vi "CAN_Write_Read_NEW.vi"(5 "Read In":refnum<k21>, 7 "Numeric Request":u32, 8 "CAN frame":T1 {"payload" format="%x"; "timestamp" format="%<%.7X\n%x>T"; "type" items=["CAN Data"=0, "CAN Remote"=1, "CAN Bus Error"=2, "CAN 2.0 Data"=8, "CAN FD Data"=16, "CAN FD+BRS Data"=24, "J1939 Data"=192, "Delay"=224, "Log Trigger"=225, "Start Trigger"=226]; "identifier" format="%x"}, 9 "Write In":refnum<k21>) -> (0 "Error Out":errorcluster, 1 "cluster":T3 {"data[0]"."payload" format="%x"; "data[0]"."timestamp" format="%<%.7X\n%x>T"; "data[0]"."type" items=["CAN Data"=0, "CAN Remote"=1, "CAN Bus Error"=2, "CAN 2.0 Data"=8, "CAN FD Data"=16, "CAN FD+BRS Data"=24, "J1939 Data"=192, "Delay"=224, "Log Trigger"=225, "Start Trigger"=226]; "data[0]"."identifier" format="%x"; "data[1]"."payload" format="%x"; "data[1]"."timestamp" format="%<%.7X\n%x>T"; "data[1]"."type" items=["CAN Data"=0, "CAN Remote"=1, "CAN Bus Error"=2, "CAN 2.0 Data"=8, "CAN FD Data"=16, "CAN FD+BRS Data"=24, "J1939 Data"=192, "Delay"=224, "Log Trigger"=225, "Start Trigger"=226]; "data[1]"."identifier" format="%x"; "data[2]"."payload" format="%x"; "data[2]"."timestamp" format="%<%.7X\n%x>T"; "data[2]"."type" items=["CAN Data"=0, "CAN Remote"=1, "CAN Bus Error"=2, "CAN 2.0 Data"=8, "CAN FD Data"=16, "CAN FD+BRS Data"=24, "J1939 Data"=192, "Delay"=224, "Log Trigger"=225, "Start Trigger"=226]; "data[2]"."identifier" format="%x"; "data[3]"."payload" format="%x"; "data[3]"."timestamp" format="%<%.7X\n%x>T"; "data[3]"."type" items=["CAN Data"=0, "CAN Remote"=1, "CAN Bus Error"=2, "CAN 2.0 Data"=8, "CAN FD Data"=16, "CAN FD+BRS Data"=24, "J1939 Data"=192, "Delay"=224, "Log Trigger"=225, "Start Trigger"=226]; "data[3]"."identifier" format="%x"; "data[4]"."payload" format="%x"; "data[4]"."timestamp" format="%<%.7X\n%x>T"; "data[4]"."type" items=["CAN Data"=0, "CAN Remote"=1, "CAN Bus Error"=2, "CAN 2.0 Data"=8, "CAN FD Data"=16, "CAN FD+BRS Data"=24, "J1939 Data"=192, "Delay"=224, "Log Trigger"=225, "Start Trigger"=226]; "data[4]"."identifier" format="%x"; "data[5]"."payload" format="%x"; "data[5]"."timestamp" format="%<%.7X\n%x>T"; "data[5]"."type" items=["CAN Data"=0, "CAN Remote"=1, "CAN Bus Error"=2, "CAN 2.0 Data"=8, "CAN FD Data"=16, "CAN FD+BRS Data"=24, "J1939 Data"=192, "Delay"=224, "Log Trigger"=225, "Start Trigger"=226]; "data[5]"."identifier" format="%x"; "data[6]"."payload" format="%x"; "data[6]"."timestamp" format="%<%.7X\n%x>T"; "data[6]"."type" items=["CAN Data"=0, "CAN Remote"=1, "CAN Bus Error"=2, "CAN 2.0 Data"=8, "CAN FD Data"=16, "CAN FD+BRS Data"=24, "J1939 Data"=192, "Delay"=224, "Log Trigger"=225, "Start Trigger"=226]; "data[6]"."identifier" format="%x"; "data[7]"."payload" format="%x"; "data[7]"."timestamp" format="%<%.7X\n%x>T"; "data[7]"."type" items=["CAN Data"=0, "CAN Remote"=1, "CAN Bus Error"=2, "CAN 2.0 Data"=8, "CAN FD Data"=16, "CAN FD+BRS Data"=24, "J1939 Data"=192, "Delay"=224, "Log Trigger"=225, "Start Trigger"=226]; "data[7]"."identifier" format="%x"; "data[8]"."payload" format="%x"; "data[8]"."timestamp" format="%<%.7X\n%x>T"; "data[8]"."type" items=["CAN Data"=0, "CAN Remote"=1, "CAN Bus Error"=2, "CAN 2.0 Data"=8, "CAN FD Data"=16, "CAN FD+BRS Data"=24, "J1939 Data"=192, "Delay"=224, "Log Trigger"=225, "Start Trigger"=226]; "data[8]"."identifier" format="%x"}, 2 "Write Out":refnum<k21>, 3 "ID Correct?":bool, 4 "Read Out":refnum<k21>)   [LabVIEW 2023]
uses:
  <vilib>/xnet/xnet.llb/XNET Frame CAN.ctl
  <vilib>/xnet/xnet.llb/XNET Frame Type CAN.ctl
panel:
  in  "Error In":errorcluster
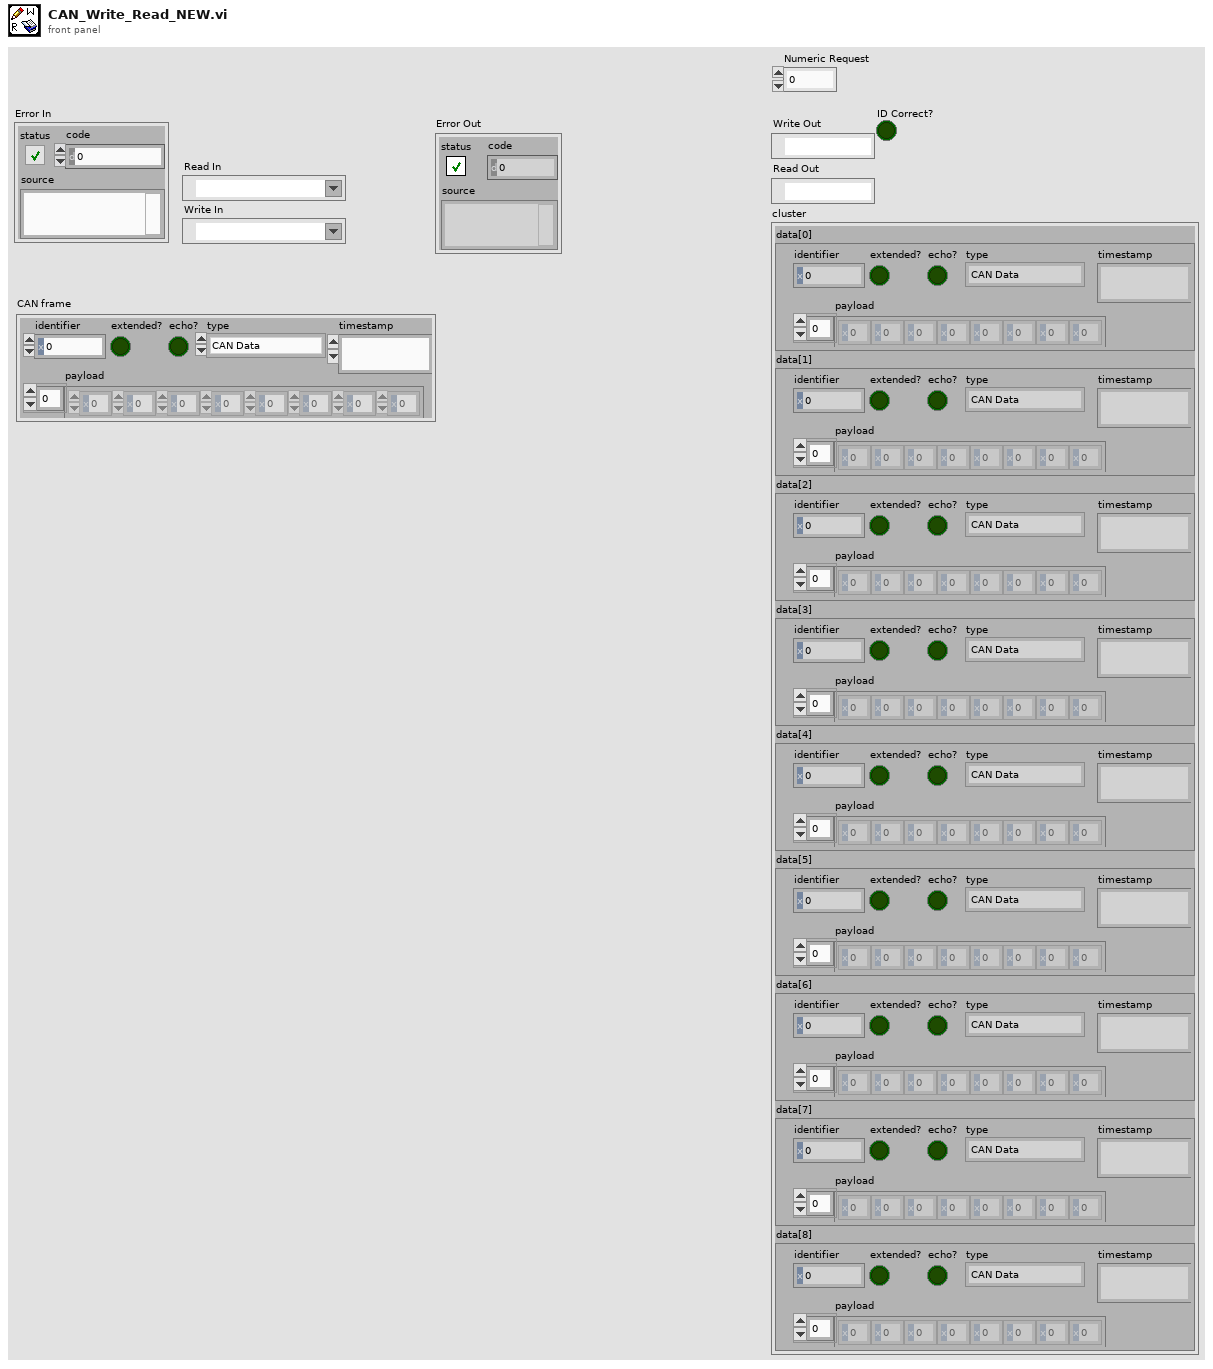
[diagram p1: front panel]
types:
  T1 = typedef "XNET Frame CAN.ctl" = cluster{"timestamp":timestamp, "payload":u8[], "identifier":u32, "type":T2, "extended?":bool, "echo?":bool}
  T2 = typedef "XNET Frame Type CAN.ctl" = u8
  T3 = cluster{"data[0]":T1, "data[1]":T1, "data[2]":T1, "data[3]":T1, "data[4]":T1, "data[5]":T1, "data[6]":T1, "data[7]":T1, "data[8]":T1}
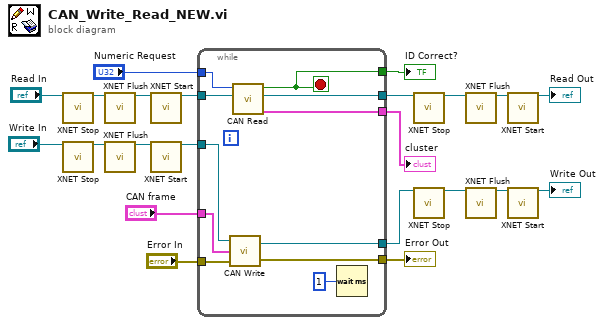
[diagram p0: block diagram]
diagram:
  n1 = call <vilib>:"XNET Stop.vi"("session in"="Read In") -> ("session out"=w21:refnum<k21>)  [unwired: 13 in, 1 out]
  n2 = call <vilib>:"XNET Stop.vi"("session in"="Write In") -> ("session out"=w16:refnum<k21>)  [unwired: 13 in, 1 out]
  n3 = call <vilib>:"XNET Flush.vi"("session in"=w21) -> ("session out"=w20:refnum<k21>)  [unwired: 13 in, 1 out]
  n4 = call <vilib>:"XNET Flush.vi"("session in"=w16) -> ("session out"=w15:refnum<k21>)  [unwired: 13 in, 1 out]
  n5 = call <vilib>:"XNET Start.vi"("session in"=w20) -> ("session out"=w19:refnum<k21>)  [unwired: 13 in, 1 out]
  n6 = call <vilib>:"XNET Start.vi"("session in"=w15) -> ("session out"=w14:refnum<k21>)  [unwired: 13 in, 1 out]
  n7 = while {
    tunnel: [w28] -> w5
    tunnel: [w29] -> w11
    tunnel: [w25] -> w10
    tunnel: [w24] -> w9
    tunnel: w19 -> [w27]
    tunnel: "Numeric Request" -> [w26]
    tunnel: w14 -> [w30]
    tunnel: "CAN frame" -> [w31]
    tunnel: "Error In" -> [w32]
    tunnel: [w23] -> w1
    stop <- w23 stop-if-true
    n8 = call "CAN Write.vi"("Error In"=w32, "CAN frame"=w31, "Write In"=w30) -> ("Error Out"=w29:errorcluster, "Write Out"=w28:refnum<k21>)
    n9 = call "CAN Read.vi"("Read In"=w27, "Numeric Request"=w26) -> ("cluster"=w25:T3, "Read Out"=w24:refnum<k21>, "ID Correct?"=w23:bool)  [unwired: 2 in, 1 out]
    n10 = Wait (ms)(milliseconds to wait=u32 1) -> ()  [unwired: 1 out]
  }
  "Error Out" <- w11
  "ID Correct?" <- w1
  "cluster" <- w10
  n11 = call <vilib>:"XNET Stop.vi"("session in"=w9) -> ("session out"=w8:refnum<k21>)  [unwired: 13 in, 1 out]
  n12 = call <vilib>:"XNET Stop.vi"("session in"=w5) -> ("session out"=w4:refnum<k21>)  [unwired: 13 in, 1 out]
  n13 = call <vilib>:"XNET Flush.vi"("session in"=w8) -> ("session out"=w7:refnum<k21>)  [unwired: 13 in, 1 out]
  n14 = call <vilib>:"XNET Flush.vi"("session in"=w4) -> ("session out"=w3:refnum<k21>)  [unwired: 13 in, 1 out]
  n15 = call <vilib>:"XNET Start.vi"("session in"=w7) -> ("session out"=→"Read Out":refnum<k21>)  [unwired: 13 in, 1 out]
  n16 = call <vilib>:"XNET Start.vi"("session in"=w3) -> ("session out"=→"Write Out":refnum<k21>)  [unwired: 13 in, 1 out]
